vi "JSONRPC-BuildInfo.vi"(6 "keywords":string, 7 "authors":string, 8 "readables":T1(array[cluster]), 9 "writables":T1(array[cluster]), 10 "description":string, 11 "expId":string) -> (3 "info":string)   [LabVIEW 2014]
panel:
  # "BuildInfo"
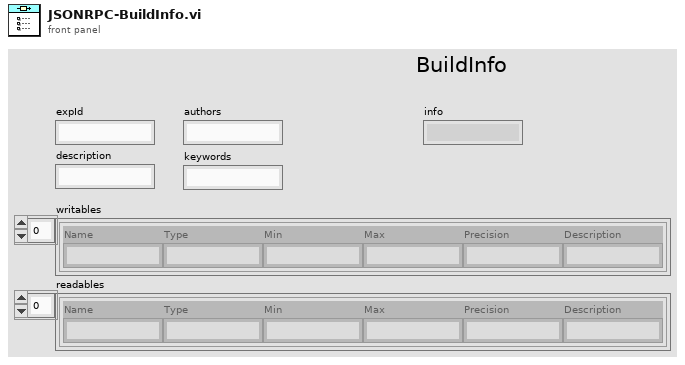
[diagram p1: front panel]
types:
  T1 = cluster{"Name":string, "Type":string, "Min":string, "Max":string, "Precision":string, "Description":string}[]
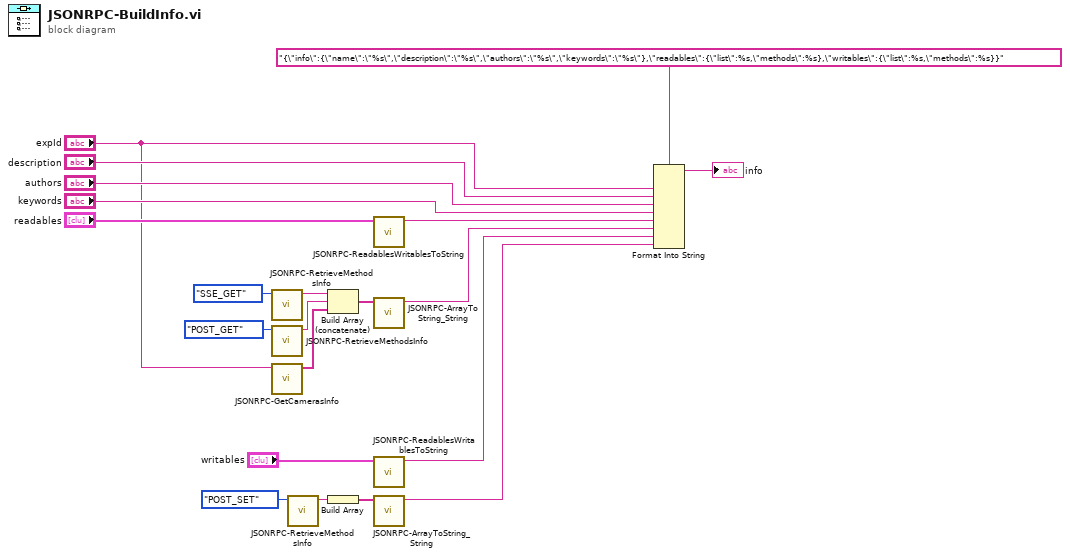
[diagram p0: block diagram]
diagram:
  n1 = call "JSONRPC-RetrieveMethodsInfo.vi"("Method"=enum16{"POST_SET", "POST_GET", "SSE_GET"}."SSE_GET") -> ("Output"=w12:string)  [unwired: 10 in]
  n2 = call "JSONRPC-RetrieveMethodsInfo.vi"("Method"=enum16{"POST_SET", "POST_GET", "SSE_GET"}."POST_GET") -> ("Output"=w13:string)  [unwired: 10 in]
  n3 = call "JSONRPC-GetCamerasInfo.vi"("expId"="expId") -> ("Output"=w2:string[])  [unwired: 10 in]
  n4 = call "JSONRPC-RetrieveMethodsInfo.vi"("Method"=enum16{"POST_SET", "POST_GET", "SSE_GET"}."POST_SET") -> ("Output"=w14:string)  [unwired: 10 in]
  n5 = Build Array (concatenate)(w12, w13, w2) -> (w8:string[])
  n6 = Build Array(w14) -> (w15:string[])
  n7 = call "JSONRPC-ReadablesWritablesToString.vi"("readables/writables"="readables") -> ("Output"=w4:string)  [unwired: 10 in]
  n8 = call "JSONRPC-ArrayToString_String.vi"("Array"=w8) -> ("Output"=w5:string)  [unwired: 10 in]
  n9 = call "JSONRPC-ReadablesWritablesToString.vi"("readables/writables"="writables") -> ("Output"=w6:string)  [unwired: 10 in]
  n10 = call "JSONRPC-ArrayToString_String.vi"("Array"=w15) -> ("Output"=w7:string)  [unwired: 10 in]
  n11 = Format Into String(format string="{\"info\":{\"name\":\"%s\",\"description\":\"%s\",\"authors\":\"%s\",\"keywords\":\"%s\"},\"readables\":{\"list\":%s,\"methods\":%s},\"writables\":{\"list\":%s,\"methods\":%s}}", "expId", "description", "authors", "keywords", w4, w5, w6, w7) -> (resulting string=→"info":string)  [unwired: 2 in, 1 out]
